vi "BuildMatrix.vi"(8 "error in (no error)":errorcluster, 11 "Evaluator in":refnum<class "Evaluator.lvclass">) -> (0 "error out":errorcluster, 2 "Array":dbl[][](array[numeric]), 3 "Evaluator out":refnum<class "Evaluator.lvclass">)   [LabVIEW 2023, in "Evaluator.lvclass"]
uses:
  Evaluator.lvclass
  Evaluator.lvclass/Evaluator.ctl
  Objective_class/Objective.lvclass
  Field_class/Field.lvclass
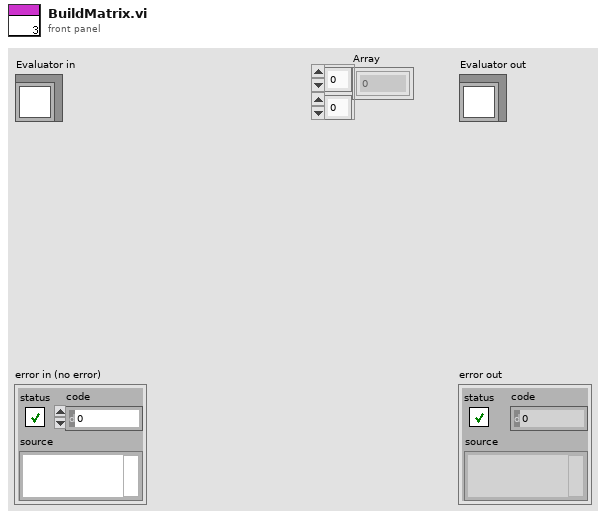
[diagram p1: front panel]
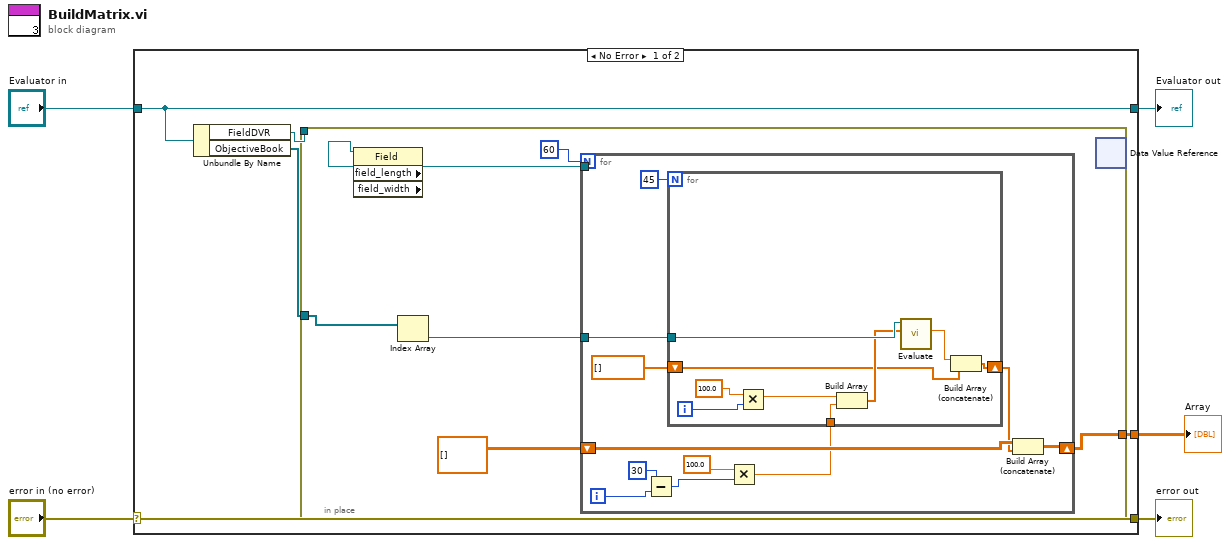
[diagram p0: block diagram]
diagram:
  n1 = case shown="No Error" "error in (no error)" {
    selector: "error in (no error)" -> [w10 w39]
    tunnel: [w10 w39] -> w4
    tunnel: [w9 w38] -> w2
    tunnel: "Evaluator in" -> [w9 w38]
    tunnel: [w6 _] -> w1
    frame No Error {
      n2 = Unbundle By Name(w9) -> ("FieldDVR"=w8:refnum<data-value>, "ObjectiveBook"=w7:refnum<class "Objective.lvclass">[])
      n3 = in-place {
        in-place-border: w8 -> [_]
        in-place-border: w7 -> [w15]
        in-place-border: [w11] -> w6
        n4 = Index Array(array=w15) -> (element=w14:refnum<class "Objective.lvclass">)  [unwired: 1 in]
        n5 = for {
          N: 60 -> [_]
          tunnel: [w28] -> w16
          tunnel: w14 -> [w27]
          shift-right: [w23] -> w11
          shift-left: dbl[][] [] ("Array") -> [w25]
          i -> [w19]
          n6 = in-place-dvr #1() -> (w28:refnum<class "Field.lvclass">)  [unwired: 1 in, 1 out]
          n7 = Subtract(x=30, y=w19) -> (x-y=w18:i32)
          n8 = Multiply(x=100.0, y=w18) -> (x*y=w17:dbl)
          n9 = for {
            N: 45 -> [_]
            tunnel: w27 -> [w37]
            shift-right: [w36] -> w24
            shift-left: dbl[] [] ("Array") -> [w30]
            tunnel: w17 -> [w32]
            i -> [w34]
            n10 = Multiply(x=100.0, y=w34) -> (x*y=w33:dbl)
            n11 = Build Array(w33, w32) -> (w31:dbl[])
            n12 = call-dynamic "Evaluate.vi"("Point"=w31, "Objective in"=w37) -> ("Evaluation"=w29:dbl)  [unwired: 7 in, 2 out]
            n13 = Build Array (concatenate)(w29, w30) -> (w36:dbl[])
          }
          n14 = Build Array (concatenate)(w25, w24) -> (w23:dbl[][])
        }
        n15 = property class="Field" props=["field_length", "field_width"](reference=w16) -> ()  [unwired: 1 in, 4 out]
        n16 = in-place-dvr #1() -> ()  [unwired: 1 in, 2 out]
      }
    }
    frame Error {
    }
  }
  "error out" <- w4
  "Evaluator out" <- w2
  "Array" <- w1
